vi "Light Meter.vi"() -> ()   [LabVIEW 2014]
doc: "This example illustrates the use of Light Meter VIs to perform intensity measurements on regions of an image. The sequence of images in this example represents an infrared view of an electronic device under test. The VI performs an intensity measurement on a rectangular area of the image to detect the overheat of a specific component."
uses:
  <vilib>/vision/NI_Vision_Development_Module.lvlib
panel:
  in  "Stop":bool
  in  "Delay (s.)":dbl(slide)=0.256 scale=0.0..0.5
  out "Intensity Chart":sgl(graph)
  out "Image Source":T1(plugin-control)
  out "Gray Level Intensities":T2 {"Standard Deviation" format="%.3f"; "Mean Intensity" format="%.3f"}
  # "Overview: Demonstrates measuring grayscale pixel intensities in a region of an image.\nRequirements: NI Vision Development Module\nInstructions: Run the VI."
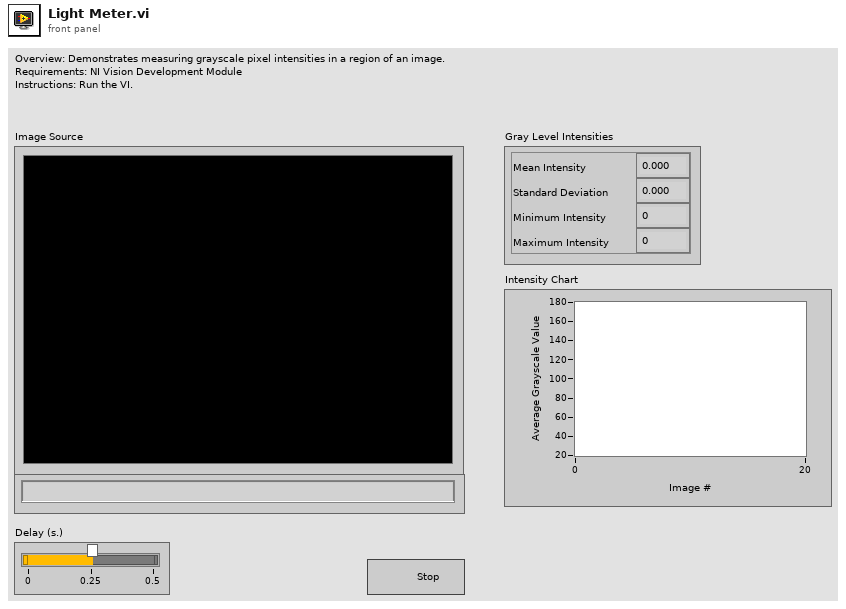
[diagram p1: front panel]
types:
  T1 = typedef "IMAQ Image.ctl" = refnum<image>
  T2 = cluster{"Mean Intensity":sgl, "Standard Deviation":sgl, "Minimum Intensity":sgl, "Maximum Intensity":sgl}
  T3 = typedef "IMAQ Rectangle" = cluster{"Left":i32, "Top":i32, "Right":i32, "Bottom":i32, "Rotation":dbl}
  T4 = cluster{"Mean Intensity":sgl, "Standard  Deviation":sgl, "Minimum Intensity":sgl, "Maximum Intensity":sgl}
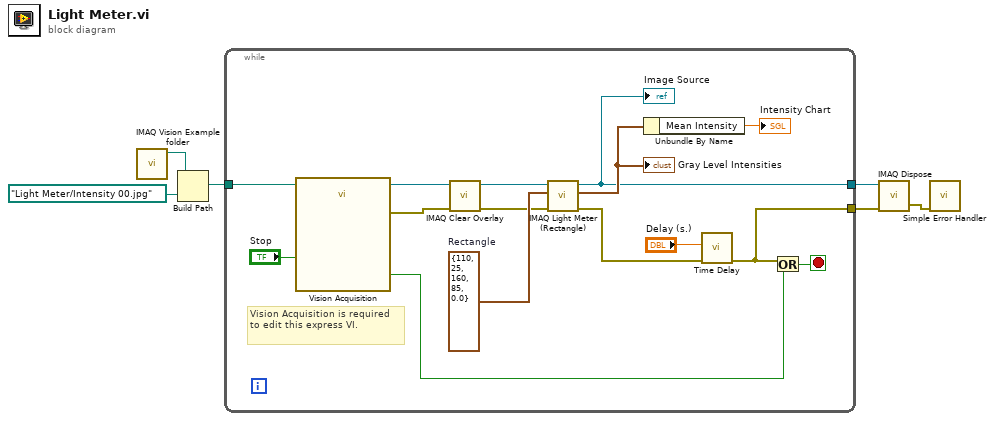
[diagram p0: block diagram]
diagram:
  n1 = call "IMAQ Vision Example folder.vi"() -> ("Example Image Path"=w6:path)  [unwired: 11 in]
  n2 = Build Path(base path=w6, name or relative path=path "Light Meter/Intensity 00.jpg") -> (appended path=w3:path)
  n3 = while {
    tunnel: w3 -> [w14]
    tunnel: [w11] -> w2
    tunnel: [w7] -> w1
    stop <- w8 stop-if-true
    w21 = T3 {"Left"=110, "Top"=25, "Right"=160, "Bottom"=85, "Rotation"=0.0}  # Rectangle
    # "Vision Acquisition is required to edit this express VI."
    n4 = call "Vision Acquisition"("Image Path"=w14, "Stop (F)"="Stop") -> ("Image Out"=w13:T1, "Stopped"=w9:bool, "error out"=w12:errorcluster)  [unwired: 23 in]
    n5 = call "IMAQ Clear Overlay"("error in (no error)"=w12, "Image"=w13) -> ("error out"=w20:errorcluster, "Image Out"=w19:T1)  [unwired: 1 in, 7 out]
    n6 = call "IMAQ Light Meter (Rectangle)"("error in (no error)"=w20, "Rectangle"=w21, "Image"=w19) -> ("error out"=w10:errorcluster, "Gray Level Intensities"=w16:T4, "Image Out"=w11:T1)  [unwired: 2 in, 4 out]
    "Gray Level Intensities" <- w16
    "Image Source" <- w11
    n7 = Unbundle By Name(w16) -> ("Mean Intensity"=→"Intensity Chart":sgl)
    n8 = call "Time Delay"("error in (no error)"=w10, "Delay Time (s)"="Delay (s.)") -> ("error out"=w7:errorcluster)  [unwired: 9 in]
    n9 = Or(x=w7, y=w9) -> (x .or. y?=w8:bool)
  }
  n10 = call "IMAQ Dispose"("Image"=w2, "error in (no error)"=w1) -> ("error out"=w4:errorcluster)  [unwired: 1 in, 3 out]
  n11 = call <vilib>:"Simple Error Handler.vi"("error in (no error)"=w4) -> ()  [unwired: 4 in, 5 out]
